vi "ilya_GetData_square.vi"(0 "adq_cu_ptr":u32, 1 "buffer_chA_in":i16[](array[numeric]), 2 "buffer_chB_in":i16[](array[numeric]), 5 "samples_per_record":u32, 7 "number_of_records":u32, 11 "error in":errorcluster) -> (4 "adq_cu_ptr":u32, 6 "function return":i32, 12 "buffer_chA_out":i16[](array[numeric]), 13 "buffer_chB_out":i16[](array[numeric]), 15 "error out":errorcluster)   [LabVIEW 2013]
uses:
  dlls/DLL_Imperium.dll
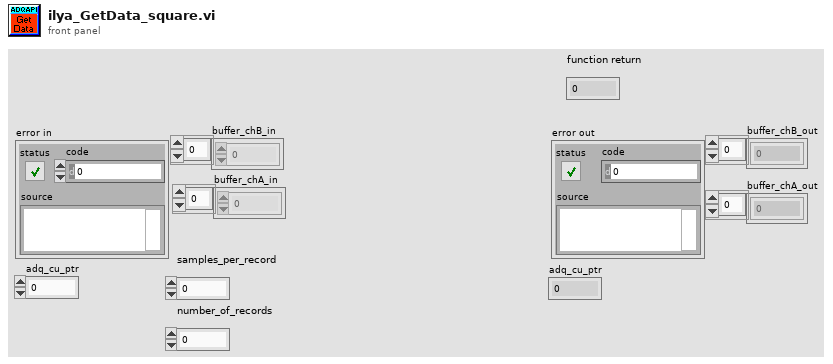
[diagram p1: front panel]
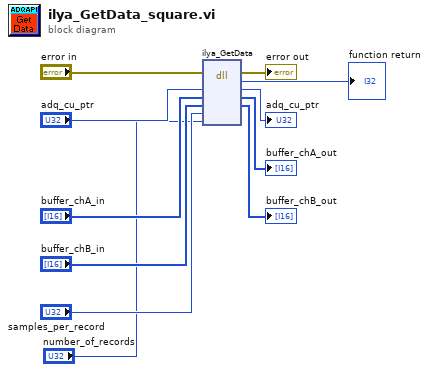
[diagram p0: block diagram]
diagram:
  n1 = dll-call lib="C:/Users/astafiev/Desktop/IlyaDrive/@photonCounting/LabView_Imperium/dlls/DLL_Imperium.dll" fn="ilya_GetData"(error in="error in", "adq_cu_ptr"="adq_cu_ptr", "buffer_chA"="buffer_chA_in", "buffer_chB"="buffer_chB_in", "samples_per_record"="samples_per_record", "number_of_records"="number_of_records") -> (error out=→"error out":errorcluster, "return type"=→"function return":i32, "adq_cu_ptr"=→"adq_cu_ptr":u32, "buffer_chA"=→"buffer_chA_out":i16[], "buffer_chB"=→"buffer_chB_out":i16[])  [unwired: 4 in, 1 out]
